vi "solar_excel Cell Next.vi"(10 "Remove Quotes? (F)":bool, 11 "Tab Delimited String in":string) -> (0 "Contain Quotes":bool, 1 "Remaining":string, 2 "Delimiter":u8, 3 "Cell out":string)   [LabVIEW 2018]
doc: "This returns the next cell from the <b>Tab Delimited String in</b> and unescapes any doule quotes (\"\")."
panel:
  # "a1\na1\\ta2\na1\\na2\n\"a1 a2\"\\t\"b2\"\n\"a1\\na2\"\\t\"b2\"\n\"a1\\n\\t\\na2\"\\t\"b2\"\na\"1\\t\"b2\"\na\"\"1\\t\"b2\"\n\"a\"\"1\"\\t\"b2\"\n\"a\"\"1\"\"\"\\t\"b2\""
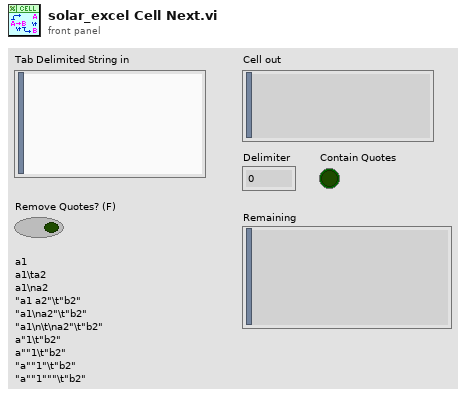
[diagram p1: front panel]
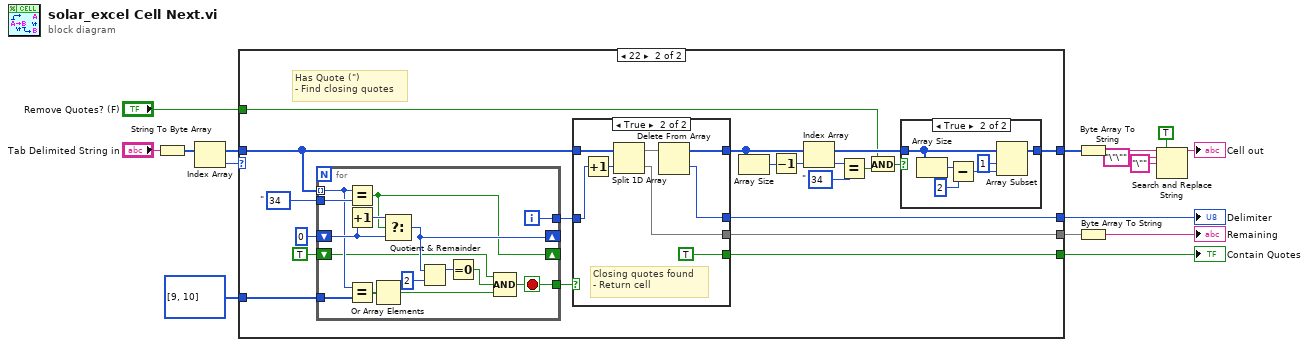
[diagram p0: block diagram]
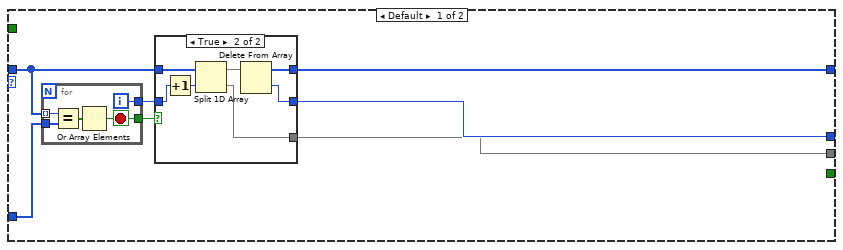
[diagram p2: hidden frame]
diagram:
  n1 = String To Byte Array(string="Tab Delimited String in") -> (unsigned byte array=w14:u8[])
  n2 = Index Array(array=w14) -> (element=w15:u8)  [unwired: 1 in]
  n3 = case shown="22" w15 {
    tunnel: w14 -> [w21 w53]
    tunnel: u8[] [9, 10] -> [w22 w54]
    tunnel: [w16 w52] -> w9
    tunnel: [w17 w51] -> w10
    tunnel: [w18 w36] -> w11
    tunnel: [_ w45] -> w8
    tunnel: "Remove Quotes? (F)" -> [_ w38]
    frame Default {
      n4 = for {
        tunnel: w21 -> [w35] mode=indexing
        tunnel: w22 -> [w34]
        tunnel: [w32] -> w19
        tunnel: [w31] -> w20
        i -> [w31]
        stop <- w32 stop-if-true
        n5 = Equal?(x=w35, y=w34) -> (x = y?=w33:bool[])
        n6 = Or Array Elements(Boolean array=w33) -> (logical OR=w32:bool)
      }
      n7 = case shown="True" w19 {
        tunnel: w20 -> [_ w30]
        tunnel: w21 -> [w23 w29]
        tunnel: [_ w26] -> w16
        tunnel: [_ w25] -> w17
        tunnel: [w23 w24] -> w18
        frame False {
        }
        frame True {
          n8 = Increment(x=w30) -> (x+1=w27:i32)
          n9 = Split 1D Array(array=w29, index=w27) -> (first subarray=w28:u8[], second subarray=w26:u8[])
          n10 = Delete From Array(array=w28) -> (deleted portion=w25:u8, array with subset deleted=w24:u8[])  [unwired: 2 in]
        }
      }
    }
    frame 34 {
      w40 = u8 34  # "
      w48 = u8 34  # "
      # "Has Quote (\")\n- Find closing quotes"
      n11 = for {
        tunnel: w53 -> [w79] mode=indexing
        tunnel: w54 -> [w85]
        tunnel: [w73] -> w50
        tunnel: [w83] -> w49
        tunnel: w48 -> [w82]
        shift-right: [w77] -> _
        shift-left: 0 -> [w80]
        shift-right: [w72] -> _
        shift-left: TRUE -> [w71]
        i -> [w83]
        stop <- w73 stop-if-true
        n12 = Equal?(x=w79, y=w82) -> (x = y?=w72:bool)
        n13 = Increment(x=w80) -> (x+1=w81:i32)
        n14 = Equal?(x=w79, y=w85) -> (x = y?=w84:bool[])
        n15 = Or Array Elements(Boolean array=w84) -> (logical OR=w74:bool)
        n16 = Select(t=w81, s=w72, f=w80) -> (s? t:f=w77:i32)
        n17 = Quotient & Remainder(x=w77, y=2) -> (x-y*floor(x/y)=w76:i32)  [unwired: 1 out]
        n18 = Equal To 0?(x=w76) -> (x = 0?=w75:bool)
        n19 = Compound Arithmetic op=AND(w71, w75, w74) -> (w73:bool)
      }
      n20 = case shown="True" w50 {
        tunnel: w49 -> [_ w70]
        tunnel: w53 -> [w62 w69]
        tunnel: [_ w66] -> w52
        tunnel: [_ w65] -> w51
        tunnel: [w62 w63] -> w44
        tunnel: [_ TRUE] -> w45
        frame False {
          # "Invalid cell format\n- Return all"
        }
        frame True {
          # "Closing quotes found\n- Return cell"
          n21 = Increment(x=w70) -> (x+1=w67:i32)
          n22 = Split 1D Array(array=w69, index=w67) -> (first subarray=w68:u8[], second subarray=w66:u8[])
          n23 = Delete From Array(array=w68) -> (deleted portion=w65:u8, array with subset deleted=w63:u8[])  [unwired: 2 in]
        }
      }
      n24 = Array Size(array=w44) -> (size(s)=w43:i32)
      n25 = Decrement(x=w43) -> (x-1=w42:i32)
      n26 = Index Array(array=w44, index=w42) -> (element=w41:u8)
      n27 = Equal?(x=w41, y=w40) -> (x = y?=w39:bool)
      n28 = And(x=w38, y=w39) -> (x .and. y?=w37:bool)
      n29 = case shown="True" w37 {
        tunnel: [w55 w61] -> w36
        tunnel: w44 -> [w55 w60]
        frame False {
          # "Keep quotes"
        }
        frame True {
          n30 = Array Size(array=w60) -> (size(s)=w58:i32)
          n31 = Subtract(x=w58, y=2) -> (x-y=w56:i32)
          n32 = Array Subset(array=w60, index=1, length=w56) -> (w61:u8[])
        }
      }
    }
  }
  "Delimiter" <- w10
  "Contain Quotes" <- w8
  n33 = Byte Array To String(unsigned byte array=w11) -> (string=w6:string)
  n34 = Byte Array To String(unsigned byte array=w9) -> (string=→"Remaining":string)
  n35 = Search and Replace String(replace all?=TRUE ("replace all? (F)"), input string=w6, search string="\"\"", replace string="\"") -> (result string=→"Cell out":string)  [unwired: 4 in, 3 out]
